vi "Get Library Classes.vi"(8 "error in (no error)":errorcluster, 11 "library ref":refnum<vi>) -> (0 "error out":errorcluster, 3 "class refs":refnum<vi>[](array[refnum]))   [LabVIEW 2017, in "Build Automation.lvlib"]
uses:
  Build Automation.lvlib
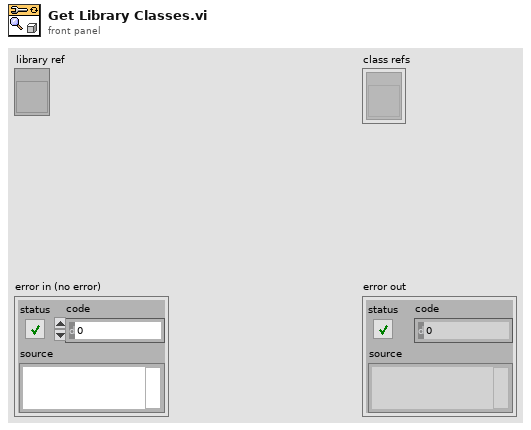
[diagram p1: front panel]
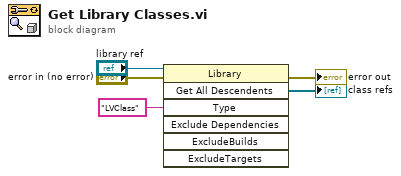
[diagram p0: block diagram]
diagram:
  n1 = invoke class="Library" method="Get All Descendents"(reference="library ref", error in="error in (no error)", "Type"="LVClass" ("y")) -> (error out=→"error out":errorcluster, "All Descendents"=→"class refs":refnum<vi>[])  [unwired: 4 in, 5 out]
